vi "GetValuesBACKUP.vi"(7 "LabVIEW Web Service Request":refnum<class "Web Request.lvclass">) -> ()   [LabVIEW 2016]
uses:
  <vilib>/wsapi/Web Request.lvclass
  <resource>/objmgr/ni.var.rc
panel:
  # "Use the Web Service Request input terminal to call the VIs on the Web Services palette. Do not remove it from the connector pane unless you don't need access to the palette."
  # "Each additional control wired to the connector pane will be available as an input in the URL. To include an indicator in terminal-mode output (the default setting), it must also be wired to the connector pane."
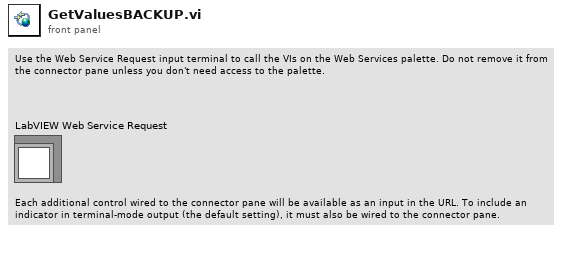
[diagram p1: front panel]
types:
  T1 = cluster{"shared variable refnum in":refnum<k21>, "shared variable refnum in 2":refnum<k21>, "shared variable refnum in 3":refnum<k21>, "shared variable refnum in 4":refnum<k21>, "shared variable refnum in 5":refnum<k21>, "shared variable refnum in 6":refnum<k21>, "shared variable refnum in 7":refnum<k21>, "shared variable refnum in 8":refnum<k21>, "shared variable refnum in 9":refnum<k21>}
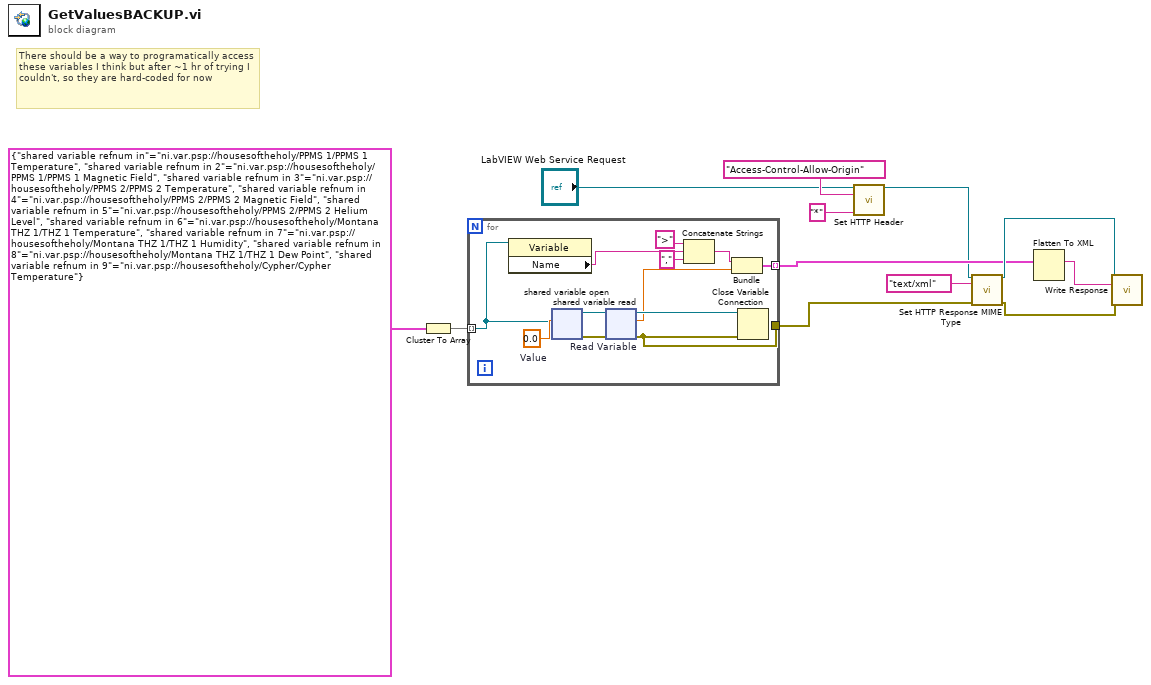
[diagram p0: block diagram]
diagram:
  # "There should be a way to programatically access these variables I think but after ~1 hr of trying I couldn't, so they are hard-coded for now"
  n1 = Cluster To Array(cluster=T1 {"shared variable refnum in"="ni.var.psp://housesoftheholy/PPMS 1/PPMS 1 Temperature", "shared variable refnum in 2"="ni.var.psp://housesoftheholy/PPMS 1/PPMS 1 Magnetic Field", "shared variable refnum in 3"="ni.var.psp://housesoftheholy/PPMS 2/PPMS 2 Temperature", "shared variable refnum in 4"="ni.var.psp://housesoftheholy/PPMS 2/PPMS 2 Magnetic Field", "shared variable refnum in 5"="ni.var.psp://housesoftheholy/PPMS 2/PPMS 2 Helium Level", "shared variable refnum in 6"="ni.var.psp://housesoftheholy/Montana THZ 1/THZ 1 Temperature", "shared variable refnum in 7"="ni.var.psp://housesoftheholy/Montana THZ 1/THZ 1 Humidity", "shared variable refnum in 8"="ni.var.psp://housesoftheholy/Montana THZ 1/THZ 1 Dew Point", "shared variable refnum in 9"="ni.var.psp://housesoftheholy/Cypher/Cypher Temperature"}) -> (array=w7:refnum<k21>[])
  n2 = for {
    tunnel: [w21] -> w9
    tunnel: w7 -> [w19] mode=indexing
    tunnel: [w18] -> w5 mode=indexing
    w20 = 0.0  # Value
    n3 = property on="Property Node" class="Variable"(reference=w19) -> ("Name"=w16:string)  [unwired: 1 in, 2 out]
    n4 = shared-variable-open(w19, w20) -> (w24:refnum<k21>, w22:errorcluster)  [unwired: 1 in]
    n5 = shared-variable-read "Read Variable"(w24, w22) -> (w23:refnum<k21>, w21:errorcluster, w17:dbl)  [unwired: 1 out]
    n6 = Concatenate Strings(">" ("string"), w16, "," ("string")) -> (w14:string)
    n7 = Bundle(w14, "Value"=w17) -> (w18:cluster{string, "Value":dbl})  [unwired: 1 in]
    n8 = Close Variable Connection(8:w21, 11:w23) -> ()  [unwired: 1 out]
  }
  n9 = call <vilib>:"Set HTTP Header.vi"("LabVIEW Web Service Request"="LabVIEW Web Service Request", "header"="Access-Control-Allow-Origin", "header value"="*") -> ("LabVIEW Web Service Request out"=w1:refnum<class "Web Request.lvclass">)  [unwired: 11 in, 1 out]
  n10 = call <vilib>:"Set HTTP Response MIME Type.vi"("LabVIEW Web Service Request"=w1, "MIME type (text/html)"="text/xml", "error in (no error)"=w9) -> ("LabVIEW Web Service Request out"=w11:refnum<class "Web Request.lvclass">, "error out"=w10:errorcluster)  [unwired: 11 in]
  n11 = Flatten To XML(anything=w5) -> (xml string=w6:string)
  n12 = call <vilib>:"Write Response.vi"("LabVIEW Web Service Request"=w11, "response string"=w6, "error in (no error)"=w10) -> ()  [unwired: 11 in, 2 out]
